vi "DriftInSDs.vi"(10 "Y":dbl[](array[numeric]), 11 "X":dbl[](array[numeric])) -> (3 "SDratioChange":dbl)   [LabVIEW 2022 SP3]
uses:
  <vilib>/Analysis/NI_AALPro.lvlib
  <vilib>/Analysis/NI_AALBase.lvlib
panel:
  # "Compares the SD of a signal with its SD if its linear trend is removed."
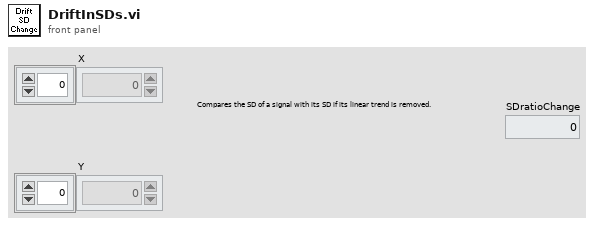
[diagram p1: front panel]
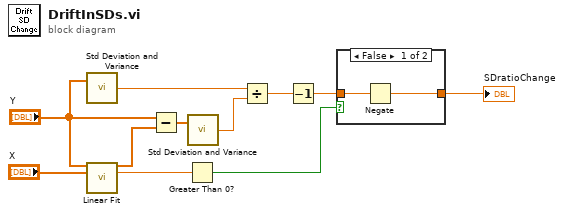
[diagram p0: block diagram]
diagram:
  n1 = call <vilib>:"Std Deviation and Variance.vi"("X"="Y") -> ("standard deviation"=w3:dbl)  [unwired: 1 in, 2 out]
  n2 = call <vilib>:"Linear Fit.vi"("Y"="Y", "X"="X") -> ("Best Linear Fit"=w1:dbl[], "slope"=w8:dbl)  [unwired: 9 in, 3 out]
  n3 = Subtract(x="Y", y=w1) -> (x-y=w2:dbl[])
  n4 = Greater Than 0?(x=w8) -> (x > 0?=w9:bool)
  n5 = call <vilib>:"Std Deviation and Variance.vi"("X"=w2) -> ("standard deviation"=w4:dbl)  [unwired: 1 in, 2 out]
  n6 = Divide(x=w3, y=w4) -> (x/y=w7:dbl)
  n7 = Decrement(x=w7) -> (x-1=w11:dbl)
  n8 = case shown="False" w9 {
    tunnel: [w12 w14] -> w10
    tunnel: w11 -> [w13 w14]
    frame False {
      n9 = Negate(x=w13) -> (-x=w12:dbl)
    }
    frame True {
    }
  }
  "SDratioChange" <- w10
